vi "Eye Scan Property Node.vi"   [LabVIEW 2014]
doc: "This property node is configured to access Eye Scan properties."
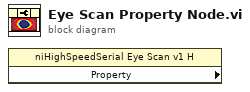
[diagram p0: block diagram]
diagram:
  n1 = property class="niHighSpeedSerial Eye Scan v1 H" props=[]() -> ()  [unwired: 2 in, 3 out]
